vi "RTEH Classification to U32.vi"(1 "Classification as String":string) -> (0 "Classification as Number":u32)   [LabVIEW 2017]
doc: "To avoid string manipulation the RTEH stores classifications as integers. This VI converts a 4 byte string into an integer for efficient transport. Strings will more than 4 characters will be truncated to 4 characters."
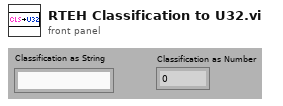
[diagram p1: front panel]
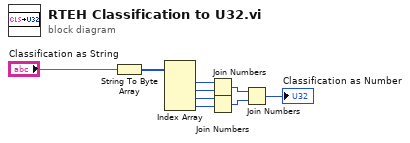
[diagram p0: block diagram]
diagram:
  n1 = String To Byte Array(string="Classification as String") -> (unsigned byte array=w8:u8[])
  n2 = Index Array(array=w8) -> (element #1=w7:u8, element #2=w6:u8, element #3=w5:u8, element #4=w4:u8)  [unwired: 4 in]
  n3 = Join Numbers(hi=w7, lo=w6) -> ((hi.lo)=w3:u16)
  n4 = Join Numbers(hi=w5, lo=w4) -> ((hi.lo)=w2:u16)
  n5 = Join Numbers(hi=w3, lo=w2) -> ((hi.lo)=→"Classification as Number":u32)
